vi "Channel.SearchForExisting.vi"(10 "Existing Channels":string[](array[string]), 11 "All Channels":string[](array[string])) -> (3 "Array out":string[](array[string]))   [LabVIEW 2013, in "Simple Sequence Tools - Editor.lvlib"]
uses:
  Simple Sequence Tools - Editor.lvlib
  Shared/Simple Sequence Tools - Shared.lvlib
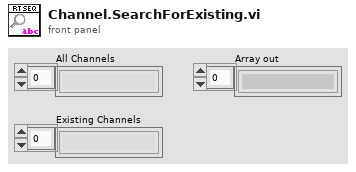
[diagram p1: front panel]
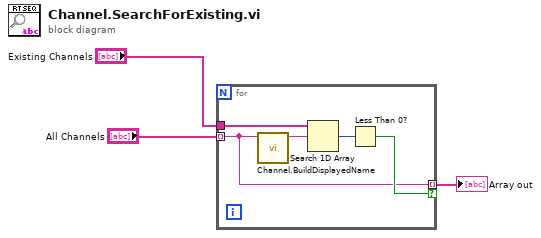
[diagram p0: block diagram]
diagram:
  n1 = for {
    tunnel: "Existing Channels" -> [w6]
    tunnel: "All Channels" -> [w5] mode=indexing
    tunnel: [w5] -> w3 mode=indexing if=w7
    n2 = call "Channel.BuildDisplayedName.vi"("Path"=w5) -> ("Formated Path"=w4:string)  [unwired: 10 in]
    n3 = Search 1D Array(1D array=w6, element=w4) -> (index of element=w8:i32)  [unwired: 1 in]
    n4 = Less Than 0?(x=w8) -> (x < 0?=w7:bool)
  }
  "Array out" <- w3
